vi "counter 1.vi"() -> ()   [LabVIEW 2010]
panel:
  out "카운트 1":i32
  out "진행 중 합계":i32
  in  "정지":bool
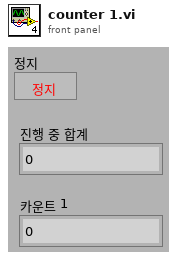
[diagram p1: front panel]
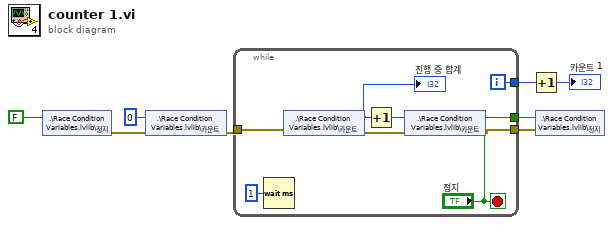
[diagram p0: block diagram]
diagram:
  n1 = shared-variable ".\\Race Condition Variables.lvlib\\정지"(FALSE ("stop")) -> (error out=w2:errorcluster)  [unwired: 1 in]
  n2 = shared-variable ".\\Race Condition Variables.lvlib\\카운트"(0 ("counter"), error in=w2) -> (error out=w8:errorcluster)
  n3 = while {
    tunnel: [w15] -> w7
    tunnel: w8 -> [w14]
    tunnel: [w10] -> w4
    tunnel: ["정지"] -> w3
    i -> [w15]
    stop <- "정지" stop-if-true
    n4 = Wait (ms)(milliseconds to wait=u32 1) -> ()  [unwired: 1 out]
    n5 = shared-variable ".\\Race Condition Variables.lvlib\\카운트"(error in=w14) -> (w11:i32, error out=w16:errorcluster)
    "진행 중 합계" <- w11
    n6 = Increment(x=w11) -> (x+1=w12:i32)
    n7 = shared-variable ".\\Race Condition Variables.lvlib\\카운트"(w12, error in=w16) -> (error out=w10:errorcluster)
  }
  n8 = Increment(x=w7) -> (x+1=→"카운트 1":i32)
  n9 = shared-variable ".\\Race Condition Variables.lvlib\\정지"(w3, error in=w4) -> ()  [unwired: 1 out]
